vi "Differential Drive Odometry.vi"(6 "Reset":bool, 9 "Theta":dbl, 10 "Right Distance":dbl, 11 "Left Distance":dbl) -> (3 "Pose":T1)   [LabVIEW 2019]
uses:
  Geometry/Typedef/Pose2d.ctl
  Geometry/Typedef/Translation2d.ctl
  Geometry/Typedef/Rotation2d.ctl
  <vilib>/Analysis/coordinate.llb/2D Cartesian Coordinate Rotation (Scalar).vi
  <vilib>/Analysis/NI_AALPro.lvlib
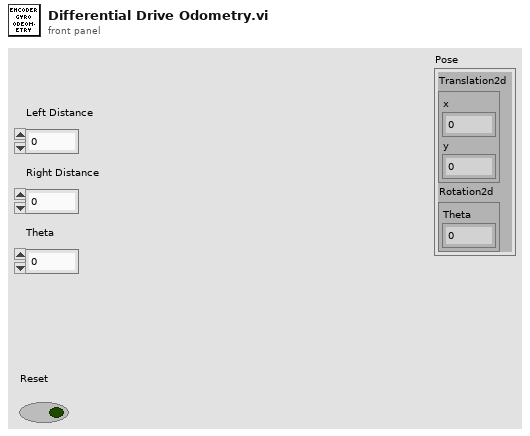
[diagram p1: front panel]
types:
  T1 = typedef "Pose2d.ctl" = cluster{"Translation2d":T2, "Rotation2d":T3}
  T2 = typedef "Translation2d.ctl" = cluster{"x":dbl, "y":dbl}
  T3 = typedef "Rotation2d.ctl" = cluster{"Theta":dbl}
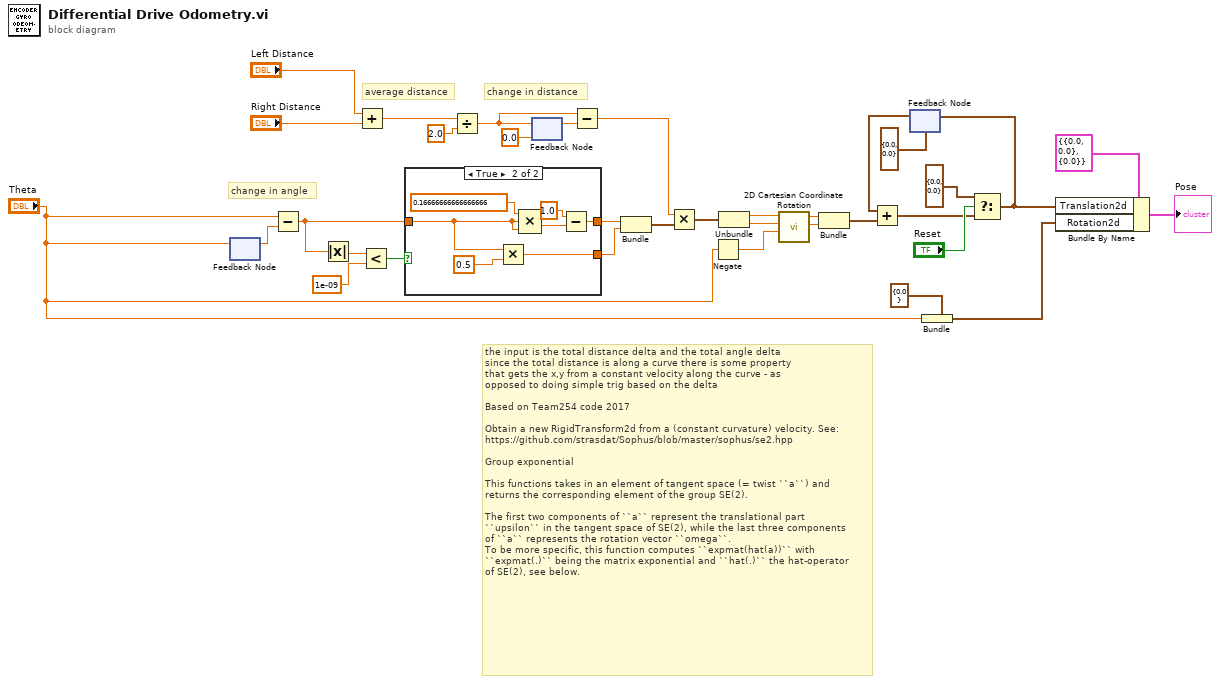
[diagram p0: block diagram]
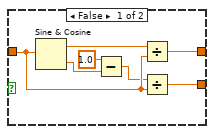
[diagram p2: hidden frame]
diagram:
  # "change in angle"
  # "the input is the total distance delta and the total angle delta\nsince the total distance is along a curve there is some property \nthat gets the x,y from a constant velocity along the curve - as\nopposed to doing simple trig based on the delta\n\nBased on Team254 code 2017\n\nObtain a new RigidTransform2d from a (constant curvature) velocity. See:\nhttps://github.com/strasdat/Sophus/blob/master/sophus/se2.hpp\n\nGroup exponential\n\nThis functions takes in an element of tangent space (= twist ``a``) and\nreturns the corresponding element of the group SE(2).\n\nThe first two components of ``a`` represent the translational part\n``upsilon`` in the tangent space of SE(2), while the last three components\nof ``a`` represents the rotation vector ``omega``.\nTo be more specific, this function computes ``expmat(hat(a))`` with\n``expmat(.)`` being the matrix exponential and ``hat(.)`` the hat-operator\nof SE(2), see below."
  # "change in distance"
  # "average distance"
  n1 = feedback-in #1("Theta") -> ()
  n2 = feedback #1() -> (w24:dbl)  [unwired: 1 in]
  n3 = Subtract(x="Theta", y=w24) -> (x-y=w20:dbl)
  n4 = Absolute Value(x=w20) -> (abs(x)=w23:dbl)
  n5 = Add(x="Left Distance", y="Right Distance") -> (x+y=w29:dbl)
  n6 = Less?(x=w23, y=1e-09) -> (x < y?=w21:bool)
  n7 = case shown="True" w21 {
    tunnel: w20 -> [w40 w42]
    tunnel: [w36 w43] -> w19
    tunnel: [w35 w47] -> w18
    frame False {
      n8 = Sine & Cosine(0:w40) -> (1:w41:dbl, 2:w38:dbl)
      n9 = Subtract(x=1.0, y=w38) -> (x-y=w37:dbl)
      n10 = Divide(x=w41, y=w40) -> (x/y=w36:dbl)
      n11 = Divide(x=w37, y=w40) -> (x/y=w35:dbl)
    }
    frame True {
      n12 = Multiply(x=w42, y=0.5) -> (x*y=w47:dbl)
      n13 = Compound Arithmetic op=MULTIPLY(0.16666666666666666 ("y"), w42, w42) -> (w46:dbl)
      n14 = Subtract(x=1.0, y=w46) -> (x-y=w43:dbl)
    }
  }
  n15 = Divide(x=w29, y=2.0) -> (x/y=w28:dbl)
  n16 = feedback #2(0.0) -> (w34:dbl)
  n17 = feedback-in #2(w28) -> ()
  n18 = Subtract(x=w28, y=w34) -> (x-y=w16:dbl)
  n19 = Bundle(w19, w18) -> (w17:cluster{dbl, dbl})  [unwired: 1 in]
  n20 = Multiply(x=w16, y=w17) -> (x*y=w15:cluster{dbl, dbl})
  n21 = Negate(x="Theta") -> (-x=w4:dbl)
  n22 = Unbundle(w15) -> (w14:dbl, w13:dbl)
  n23 = call-poly <vilib>:"2D Cartesian Coordinate Rotation.vi"("theta"=w4, "y"=w13, "x"=w14) -> ("y out"=w11:dbl, "x out"=w12:dbl)  [unwired: 6 in, 1 out]
  n24 = Bundle("x out"=w12, "y out"=w11) -> (w10:cluster{"x out":dbl, "y out":dbl})  [unwired: 1 in]
  n25 = feedback #3(T2 {"x"=0.0, "y"=0.0} ("Translation2d")) -> (w32:T2)
  n26 = Add(x=w32, y=w10) -> (x+y=w25:T2)
  n27 = Bundle(cluster=T3 {"Theta"=0.0} ("Rotation2d"), "Theta"="Theta") -> (w2:T3)
  n28 = Select(t=T2 {"x"=0.0, "y"=0.0} ("Translation2d"), s="Reset", f=w25) -> (s? t:f=w5:T2)
  n29 = feedback-in #3(w5) -> ()
  n30 = Bundle By Name(cluster=T1 {"Translation2d"={"x"=0.0, "y"=0.0}, "Rotation2d"={"Theta"=0.0}} ("Pose2d"), "Translation2d"=w5, "Rotation2d"=w2) -> (→"Pose":T1)
